vi "_Calculate ADC Value.vi"(0 "ADC Values":i32[](array[numeric]), 1 "ADC Channel (64)":u8) -> (2 "User Value":sgl, 3 "In Range?":bool, 4 "Raw Reading":sgl)   [LabVIEW 2012]
uses:
  _RT Global.vi
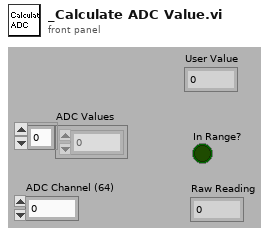
[diagram p1: front panel]
types:
  T1 = typedef "_RT Configuration 2.ctl" = cluster{"Name":string, "Ch#":u8, "Min":dbl, "Max":dbl, "Def+":dbl, "Def-":dbl, "Offset":dbl, "Slope":dbl, "Type":u8, "Description":string, "SettleT":dbl}
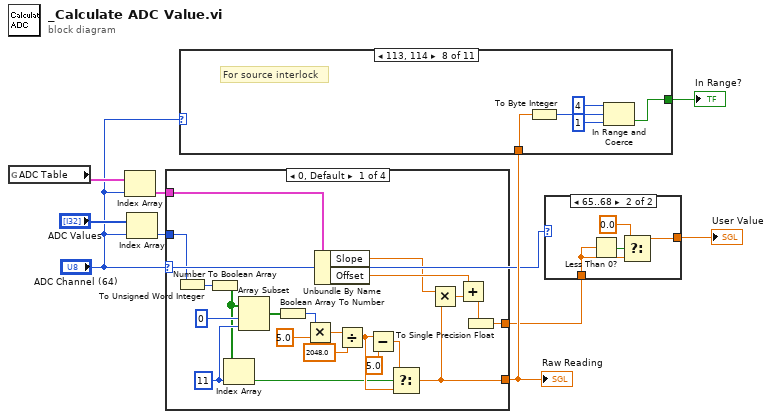
[diagram p0: block diagram]
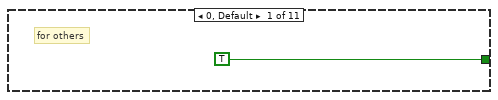
[diagram p3: hidden frame]
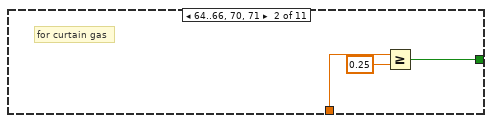
[diagram p4: hidden frame]
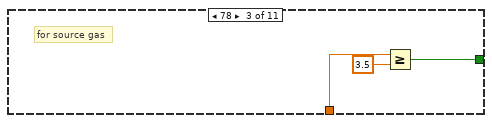
[diagram p5: hidden frame]
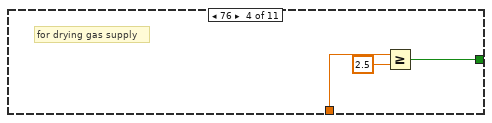
[diagram p6: hidden frame]
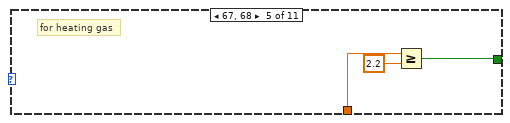
[diagram p7: hidden frame]
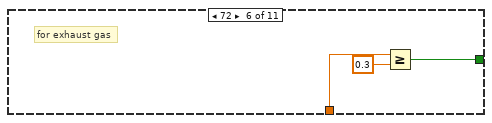
[diagram p8: hidden frame]
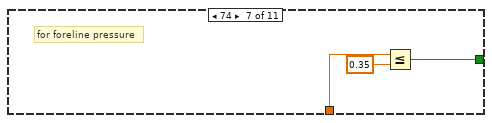
[diagram p9: hidden frame]
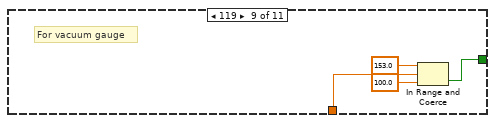
[diagram p10: hidden frame]
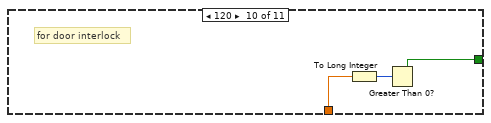
[diagram p11: hidden frame]
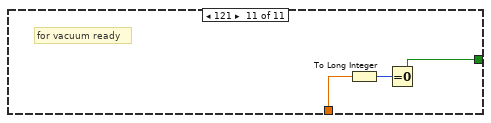
[diagram p12: hidden frame]
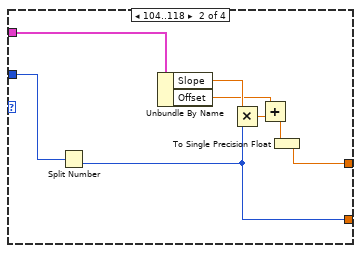
[diagram p13: hidden frame]
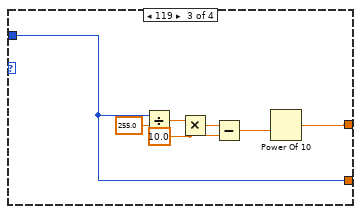
[diagram p14: hidden frame]
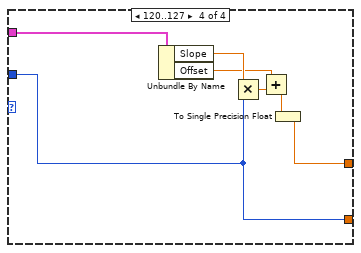
[diagram p15: hidden frame]
diagram:
  n1 = global read "_RT Global.vi" "ADC Table"() -> (w7:T1[])
  n2 = Index Array(array=w7, index="ADC Channel (64)") -> (element=w6:T1)
  n3 = Index Array(array="ADC Values", index="ADC Channel (64)") -> (element=w8:i32)
  n4 = case shown="0, Default" "ADC Channel (64)" {
    tunnel: [w13 w33 w40 w48] -> w4
    tunnel: w8 -> [w17 w38 w40 w48]
    tunnel: [w11 w32 w39 w47] -> w2
    tunnel: w6 -> [w10 w31 _ w46]
    frame 0, Default {
      w19 = 11 ("index")
      n5 = To Unsigned Word Integer(number=w17) -> (unsigned 16bit integer=w27:u16)
      n6 = Number To Boolean Array(number=w27) -> (Boolean array=w18:bool[])
      n7 = Index Array(array=w18, index=w19) -> (element=w24:bool)
      n8 = Array Subset(array=w18, index=0, length=w19) -> (w20:bool[])
      n9 = Boolean Array To Number(Boolean array=w20) -> (number=w23:u32)
      n10 = Multiply(x=w23, y=sgl 5.0) -> (x*y=w28:sgl)
      n11 = Unbundle By Name(w10) -> ("Slope"=w14:dbl, "Offset"=w15:dbl)
      n12 = Divide(x=w28, y=sgl 2048.0) -> (x/y=w30:sgl)
      n13 = Subtract(x=w30, y=sgl 5.0) -> (x-y=w26:sgl)
      n14 = Select(t=w26, s=w24, f=w30) -> (s? t:f=w13:sgl)
      n15 = Multiply(x=w14, y=w13) -> (x*y=w16:dbl)
      n16 = Add(x=w15, y=w16) -> (x+y=w12:dbl)
      n17 = To Single Precision Float(number=w12) -> (single precision float=w11:sgl)
    }
    frame 104..118 {
      n18 = Split Number(x=w38) -> (lo(x)=w33:u16)  [unwired: 1 out]
      n19 = Unbundle By Name(w31) -> ("Slope"=w35:dbl, "Offset"=w34:dbl)
      n20 = Multiply(x=w35, y=w33) -> (x*y=w37:dbl)
      n21 = Add(x=w34, y=w37) -> (x+y=w36:dbl)
      n22 = To Single Precision Float(number=w36) -> (single precision float=w32:sgl)
    }
    frame 119 {
      w41 = sgl 10.0 ("y")
      n23 = Divide(x=w40, y=sgl 255.0) -> (x/y=w44:sgl)
      n24 = Multiply(x=w44, y=w41) -> (x*y=w43:sgl)
      n25 = Subtract(x=w43, y=w41) -> (x-y=w42:sgl)
      n26 = Power Of 10(x=w42) -> (10^x=w39:sgl)
    }
    frame 120..127 {
      n27 = Unbundle By Name(w46) -> ("Slope"=w50:dbl, "Offset"=w49:dbl)
      n28 = Multiply(x=w50, y=w48) -> (x*y=w52:dbl)
      n29 = Add(x=w49, y=w52) -> (x+y=w51:dbl)
      n30 = To Single Precision Float(number=w51) -> (single precision float=w47:sgl)
    }
  }
  "Raw Reading" <- w4
  n31 = case shown="113, 114" "ADC Channel (64)" {
    tunnel: [TRUE w54 w57 w60 w64 w66 w69 w72 w78 w81 w84] -> w5
    tunnel: w4 -> [_ w56 w59 w62 w65 w68 w71 w76 w77 w82 w85]
    frame 0, Default {
      # "for others"
    }
    frame 64..66, 70, 71 {
      # "for curtain gas"
      n32 = Greater Or Equal?(x=w56, y=0.25) -> (x >= y?=w54:bool)
    }
    frame 78 {
      # "for source gas"
      n33 = Greater Or Equal?(x=w59, y=3.5) -> (x >= y?=w57:bool)
    }
    frame 76 {
      # "for drying gas supply"
      n34 = Greater Or Equal?(x=w62, y=2.5) -> (x >= y?=w60:bool)
    }
    frame 67, 68 {
      # "for heating gas"
      n35 = Greater Or Equal?(x=w65, y=2.2) -> (x >= y?=w64:bool)
    }
    frame 72 {
      # "for exhaust gas"
      n36 = Greater Or Equal?(x=w68, y=0.3) -> (x >= y?=w66:bool)
    }
    frame 74 {
      # "for foreline pressure"
      n37 = Less Or Equal?(x=w71, y=0.35) -> (x <= y?=w69:bool)
    }
    frame 113, 114 {
      # "For source interlock"
      n38 = To Byte Integer(number=w76) -> (8bit integer=w73:i8)
      n39 = In Range and Coerce(upper limit=i8 4, x=w73, lower limit=i8 1) -> (In Range?=w72:bool)  [unwired: 1 out]
    }
    frame 119 {
      # "For vacuum gauge"
      n40 = In Range and Coerce(upper limit=sgl 153.0, x=w77, lower limit=sgl 100.0) -> (In Range?=w78:bool)  [unwired: 1 out]
    }
    frame 120 {
      # "for door interlock"
      n41 = To Long Integer(number=w82) -> (32bit integer=w83:i32)
      n42 = Greater Than 0?(x=w83) -> (x > 0?=w81:bool)
    }
    frame 121 {
      # "for vacuum ready"
      n43 = To Long Integer(number=w85) -> (32bit integer=w86:i32)
      n44 = Equal To 0?(x=w86) -> (x = 0?=w84:bool)
    }
  }
  "In Range?" <- w5
  n45 = case shown="65..68" "ADC Channel (64)" {
    tunnel: w2 -> [w87 w90]
    tunnel: [w87 w89] -> w1
    frame 0, Default {
    }
    frame 65..68 {
      n46 = Less Than 0?(x=w90) -> (x < 0?=w91:bool)
      n47 = Select(t=sgl 0.0, s=w91, f=w90) -> (s? t:f=w89:sgl)
    }
  }
  "User Value" <- w1
